vi "Get Dqmh Module Info.vi"(7 "Config":refnum<class "TAF Proj Config.lvclass">, 8 "error in":errorcluster, 11 "Library Ref":refnum<vi>) -> (0 "error out":errorcluster, 3 "Dqmh Module Info":T1={"Name"="", "Description"="", "Path"=path "", "Dqmh Module Type"=enum."Singleton", "Event Info"=[], "Start Module Info"={"Vi Path"=path "", "Name"="", "Description"="", "Event Type"=enum."Request", "Callers"=[], "Conpane Image"={"image type"=0, "image depth"=0, "image"=[], "mask"=[], "colors"=[], "Rectangle"={"left"=0, "top"=0, "right"=0, "bottom"=0}}}, "Stop Module Info"={"Vi Path"=path "", "Name"="", "Description"="", "Event Type"=enum."Request", "Callers"=[], "Conpane Image"={"image type"=0, "image depth"=0, "image"=[], "mask"=[], "colors"=[], "Rectangle"={"left"=0, "top"=0, "right"=0, "bottom"=0}}}, "Registred Broadcast"=[], "Custom Errors"=[], "Used Requests"=[], "Used Requests With Reply"=[]})   [LabVIEW 2021, in "TAF Proj Document Type.lvlib" / "Project Parser.lvlib"]
uses:
  <vilib>/Wovalab/AntiDoc/Document Type/Add-ons/LabVIEW TAF Project/Project Parser/Project Parser.lvlib
  <vilib>/Wovalab/AntiDoc/Document Type/Add-ons/LabVIEW TAF Project/Project Parser/Dqmh Module Info--cluster.ctl
  <vilib>/Wovalab/AntiDoc/Document Type/Add-ons/LabVIEW TAF Project/Project Parser/Dqmh Module Type--enum.ctl
  <vilib>/Wovalab/AntiDoc/Document Type/Add-ons/LabVIEW TAF Project/Project Parser/Dqmh Event Info--cluster.ctl
  <vilib>/Wovalab/AntiDoc/Document Type/Add-ons/LabVIEW TAF Project/Project Parser/Dqmh Event Type--enum.ctl
  <vilib>/Wovalab/AntiDoc/Document Type/Add-ons/LabVIEW TAF Project/Project Parser/Dqmh Event Links--cluster.ctl
  <vilib>/picture/picture.llb/imagedata.ctl
  <vilib>/Wovalab/AntiDoc/Document Type/Add-ons/LabVIEW TAF Project/Project Parser/Module Fonctions--cluster.ctl
  <vilib>/Wovalab/AntiDoc/Document Type/Add-ons/LabVIEW TAF Project/Project Parser/Custom Error Info.ctl
  <vilib>/Wovalab/AntiDoc/Document Type/Add-ons/LabVIEW TAF Project/Dqmh Module/Requests Used By Module--cluster.ctl
  <vilib>/Wovalab/AntiDoc/Document Type/Add-ons/LabVIEW TAF Project/TAF Proj Config/TAF Proj Config.lvclass
  <vilib>/Wovalab/AntiDoc/Document Type/Add-ons/LabVIEW TAF Project/Project Parser/Module Fonctions--enum.ctl
  <vilib>/Wovalab/AntiDoc/Document Type/Add-ons/LabVIEW TAF Project/Dqmh Module/Dqmh Module.lvclass
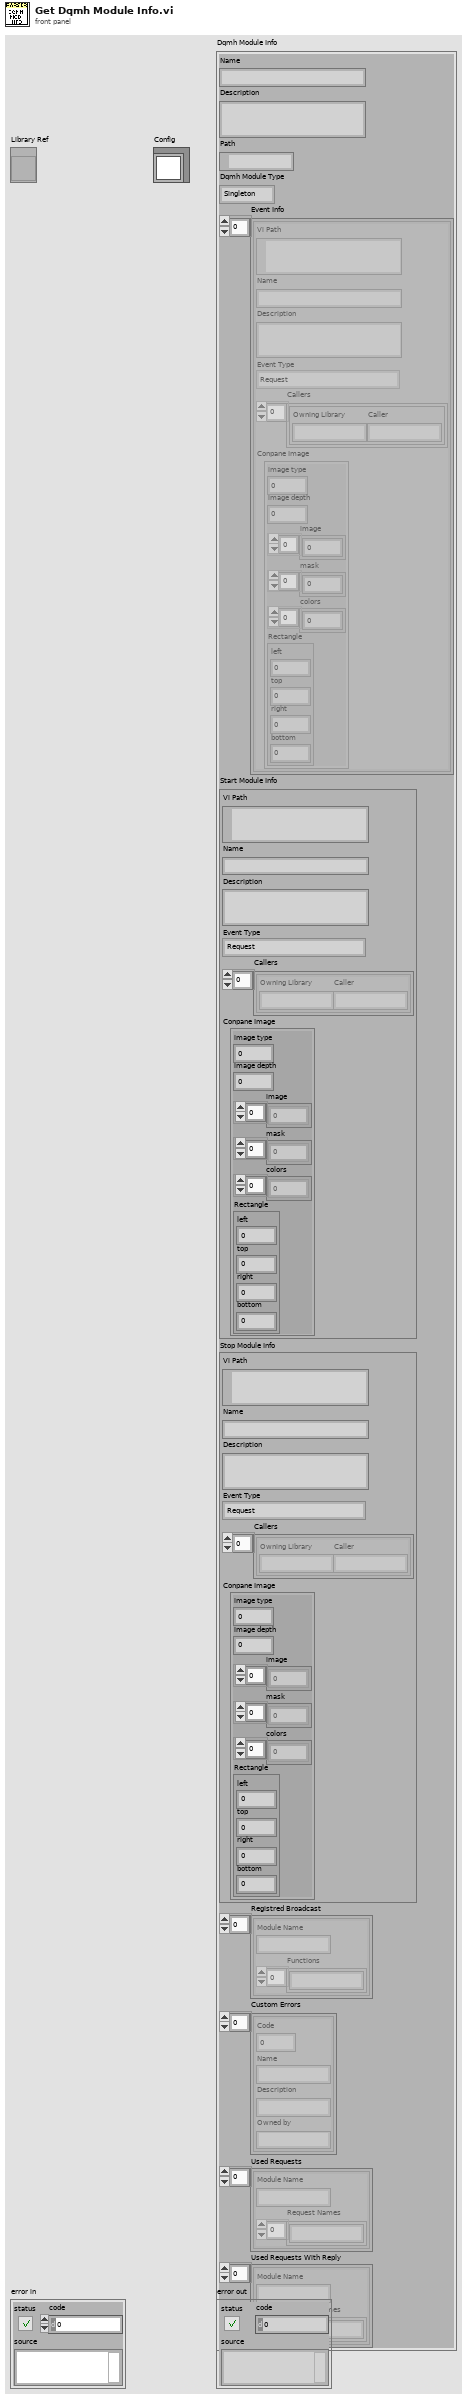
[diagram p1: front panel]
types:
  T1 = typedef "TAF Proj Document Type.lvlib/Project Parser.lvlib/Dqmh Module Info--cluster.ctl" = cluster{"Name":string, "Description":string, "Path":path, "Dqmh Module Type":T2, "Event Info":T3[], "Start Module Info":T3, "Stop Module Info":T3, "Registred Broadcast":T7[], "Custom Errors":T8[], "Used Requests":T9[], "Used Requests With Reply":T9[]}
  T2 = typedef "TAF Proj Document Type.lvlib/Project Parser.lvlib/Dqmh Module Type--enum.ctl" = enum16{"Singleton", "Cloneable"}
  T3 = typedef "TAF Proj Document Type.lvlib/Project Parser.lvlib/Dqmh Event Info--cluster.ctl" = cluster{"Vi Path":path, "Name":string, "Description":string, "Event Type":T4, "Callers":T5[], "Conpane Image":T6}
  T4 = typedef "TAF Proj Document Type.lvlib/Project Parser.lvlib/Dqmh Event Type--enum.ctl" = enum16{"Not a DQMH Event", "Request", "Request And Wait For Reply", "Broadcast"}
  T5 = typedef "TAF Proj Document Type.lvlib/Project Parser.lvlib/Dqmh Event Links--cluster.ctl" = cluster{"Owning Library":string, "Caller":string}
  T6 = typedef "imagedata.ctl" = cluster{"image type":i32, "image depth":i32, "image":u8[], "mask":u8[], "colors":u32[], "Rectangle":cluster{"left":i16, "top":i16, "right":i16, "bottom":i16}}
  T7 = typedef "TAF Proj Document Type.lvlib/Project Parser.lvlib/Module Fonctions--cluster.ctl" = cluster{"Module Name":string, "Functions":string[]}
  T8 = typedef "TAF Proj Document Type.lvlib/Project Parser.lvlib/Custom Error Info.ctl" = cluster{"Code":i32, "Name":string, "Description":string, "Owned by":string}
  T9 = typedef "TAF Proj Document Type.lvlib/Dqmh Module.lvclass/Requests Used By Module--cluster.ctl" = cluster{"Module Name":string, "Request Names":string[]}
  T10 = typedef "TAF Proj Document Type.lvlib/Project Parser.lvlib/Module Fonctions--enum.ctl" = enum16{"Event Registration", "Request"}
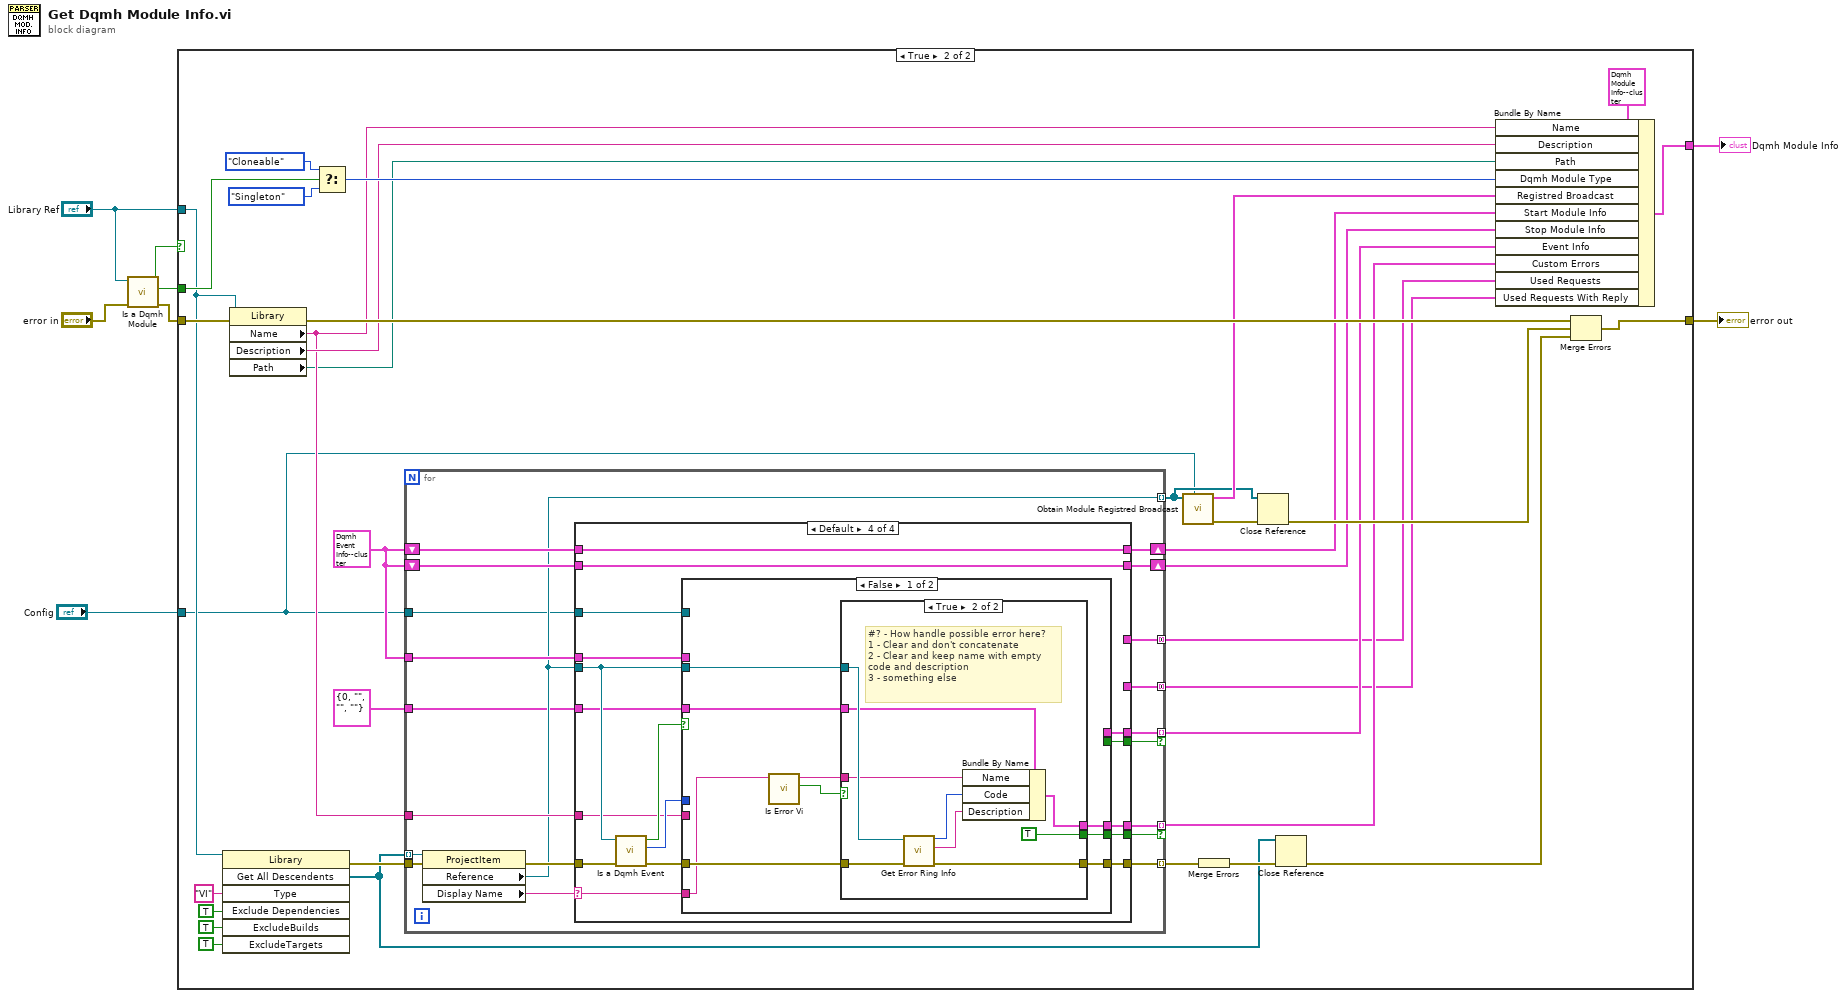
[diagram p0: block diagram]
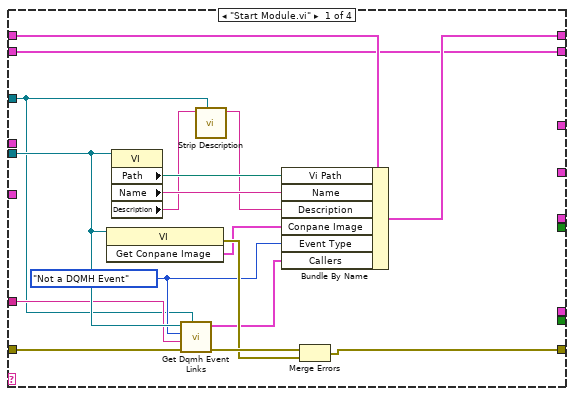
[diagram p3: hidden frame]
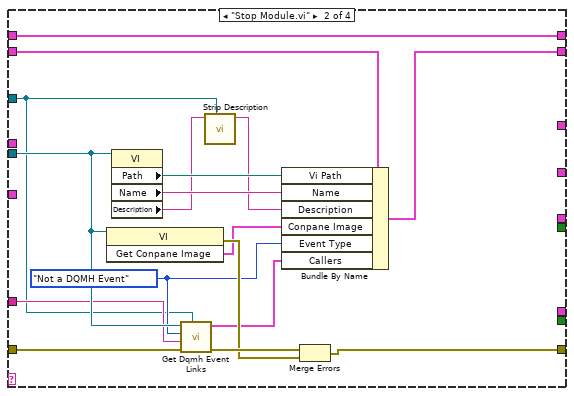
[diagram p4: hidden frame]
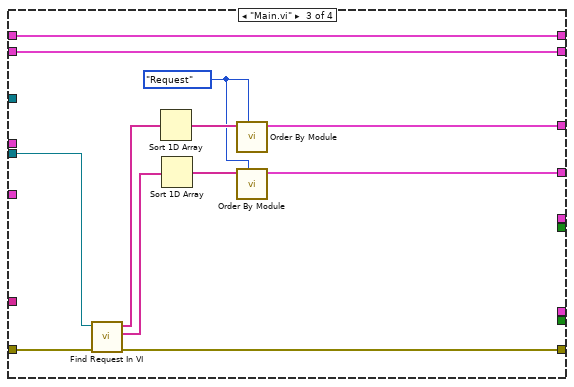
[diagram p5: hidden frame]
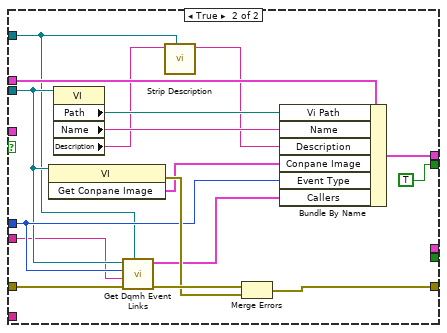
[diagram p7: hidden frame]
diagram:
  n1 = call <vilib>:"Is a Dqmh Module.vi"("error in"="error in", "Library Ref"="Library Ref") -> ("error out"=w6:errorcluster, "Is Cloneable"=w4:bool, "Is Dqmh Module"=w2:bool)  [unwired: 7 in]
  n2 = case shown="True" w2 {
    tunnel: [_ w35] -> w5
    tunnel: w4 -> [_ w34]
    tunnel: "Library Ref" -> [_ w29]
    tunnel: [w9 w41] -> w7
    tunnel: w6 -> [w9 w44]
    tunnel: "Config" -> [_ w12]
    frame False {
    }
    frame True {
      w21 = T3 {"Vi Path"=path "", "Name"="", "Description"="", "Event Type"=enum."Not a DQMH Event", "Callers"=[], "Conpane Image"={"image type"=0, "image depth"=0, "image"=[], "mask"=[], "colors"=[], "Rectangle"={"left"=0, "top"=0, "right"=0, "bottom"=0}}} ("Dqmh Event Info")
      n3 = invoke class="Library" method="Get All Descendents"(reference=w29, "Type"="VI", "Exclude Dependencies"=TRUE ("ExcludeDependencies"), "ExcludeBuilds"=TRUE, "ExcludeTargets"=TRUE) -> (error out=w43:errorcluster, "All Descendents"=w13:refnum<vi>[])  [unwired: 2 in, 5 out]
      n4 = property class="Library"(reference=w29, error in=w44) -> (error out=w42:errorcluster, "Name"=w22:string, "Description"=w30:string, "Path"=w17:path)  [unwired: 1 out]
      n5 = Select(t=Dqmh_Module_Type--enum."Cloneable" ("Dqmh Module Type"), s=w34, f=Dqmh_Module_Type--enum."Singleton") -> (s? t:f=w32:T2)
      n6 = for {
        tunnel: w13 -> [w58] mode=indexing
        tunnel: w21 -> [w61]
        tunnel: [w60] -> w27 mode=indexing if=w59
        tunnel: w43 -> [w63]
        tunnel: [w62] -> w26 mode=indexing
        tunnel: w22 -> [w57]
        shift-right: [w53] -> w19
        shift-left: w21 -> [w52]
        shift-right: [w55] -> w20
        shift-left: w21 -> [w54]
        tunnel: [w51] -> w14 mode=indexing
        tunnel: T8 {"Code"=0, "Name"="", "Description"="", "Owned by"=""} ("Custom Error Info") -> [w50]
        tunnel: [w49] -> w15 mode=indexing if=w48
        tunnel: w12 -> [w47]
        tunnel: [w46] -> w11 mode=concatenating
        tunnel: [w45] -> w10 mode=concatenating
        n7 = property class="ProjectItem"(reference=w58, error in=w63) -> (error out=w64:errorcluster, "Reference"=w51:refnum<vi>, "Display Name"=w56:string)  [unwired: 1 out]
        n8 = case shown="Default" w56 {
          selector: w56 -> [_ _ _ w115]
          tunnel: w64 -> [w79 w96 w106 w127]
          tunnel: [w78 w95 w107 w125] -> w62
          tunnel: w61 -> [_ _ _ w124]
          tunnel: [_ _ _ w121] -> w60
          tunnel: [_ _ _ w120] -> w59
          tunnel: w51 -> [w76 w94 w108 w119]
          tunnel: w57 -> [w71 w90 _ w118]
          tunnel: w54 -> [w77 w86 w110 w116]
          tunnel: [w72 w86 w110 w116] -> w55
          tunnel: [w69 w87 w109 w117] -> w53
          tunnel: w52 -> [w69 w88 w109 w117]
          tunnel: w50 -> [_ _ _ w114]
          tunnel: [_ _ _ w113] -> w49
          tunnel: [_ _ _ w112] -> w48
          tunnel: w47 -> [w65 w82 _ w111]
          tunnel: [_ _ w100 _] -> w46
          tunnel: [_ _ w99 _] -> w45
          frame "Start Module.vi" {
            w70 = Dqmh_Event_Type--enum."Not a DQMH Event" ("Event Type")
            n9 = invoke class="VI" method="Get Conpane Image"(reference=w76) -> (error out=w80:errorcluster, "Get Conpane Image"=w73:T6)  [unwired: 2 in, 1 out]
            n10 = property class="VI"(reference=w76) -> ("Path"=w75:path, "Name"=w68:string, "Description"=w67:string)  [unwired: 1 in, 2 out]
            n11 = call <vilib>:"Get Dqmh Event Links.vi"("Config"=w65, "error in"=w79, "Module Name"=w71, "Event Type"=w70, "VI Refnum"=w76) -> ("error out"=w81:errorcluster, "Links"=w74:T5[])  [unwired: 5 in]
            n12 = call <vilib>:"Strip Description.vi"("Config"=w65, "Description in"=w67) -> ("Description out"=w66:string)  [unwired: 9 in]
            n13 = Bundle By Name(cluster=w77, "Vi Path"=w75, "Name"=w68, "Description"=w66, "Conpane Image"=w73, "Event Type"=w70, "Callers"=w74) -> (w72:T3)
            n14 = Merge Errors(w81, w80) -> (w78:errorcluster)
          }
          frame "Stop Module.vi" {
            w89 = Dqmh_Event_Type--enum."Not a DQMH Event" ("Event Type")
            n15 = invoke class="VI" method="Get Conpane Image"(reference=w94) -> (error out=w97:errorcluster, "Get Conpane Image"=w91:T6)  [unwired: 2 in, 1 out]
            n16 = property class="VI"(reference=w94) -> ("Path"=w93:path, "Name"=w85:string, "Description"=w84:string)  [unwired: 1 in, 2 out]
            n17 = call <vilib>:"Get Dqmh Event Links.vi"("Config"=w82, "error in"=w96, "Module Name"=w90, "Event Type"=w89, "VI Refnum"=w94) -> ("error out"=w98:errorcluster, "Links"=w92:T5[])  [unwired: 5 in]
            n18 = call <vilib>:"Strip Description.vi"("Config"=w82, "Description in"=w84) -> ("Description out"=w83:string)  [unwired: 9 in]
            n19 = Bundle By Name(cluster=w88, "Vi Path"=w93, "Name"=w85, "Description"=w83, "Conpane Image"=w91, "Event Type"=w89, "Callers"=w92) -> (w87:T3)
            n20 = Merge Errors(w98, w97) -> (w95:errorcluster)
          }
          frame "Main.vi" {
            w101 = Module_Fonctions--enum."Request" ("Mode")
            n21 = call <vilib>:"Find Request In VI.vi"("error in"=w106, "VI Ref"=w108) -> ("error out"=w107:errorcluster, "Request And Wait For Reply Names"=w103:string[], "Request Names"=w105:string[])  [unwired: 6 in, 1 out]
            n22 = Sort 1D Array(array=w105) -> (sorted array=w104:string[])
            n23 = Sort 1D Array(array=w103) -> (sorted array=w102:string[])
            n24 = call <vilib>:"Order By Module.vi"("Mode"=w101, "Functions"=w104) -> ("Functions by Module"=w100:T7[])  [unwired: 9 in]
            n25 = call <vilib>:"Order By Module.vi"("Mode"=w101, "Functions"=w102) -> ("Functions by Module"=w99:T7[])  [unwired: 9 in]
          }
          frame Default {
            n26 = call <vilib>:"Is a Dqmh Event.vi"("error in"=w127, "VI Refnum"=w119) -> ("error out"=w126:errorcluster, "Event Type"=w123:T4, "Is Dqmh Event"=w122:bool)  [unwired: 7 in]
            n27 = case shown="False" w122 {
              tunnel: w124 -> [_ w159]
              tunnel: w123 -> [_ w154]
              tunnel: w119 -> [w132 w153]
              tunnel: [_ w157] -> w121
              tunnel: [_ TRUE] -> w120
              tunnel: w126 -> [w135 w163]
              tunnel: [w136 w161] -> w125
              tunnel: w118 -> [_ w151]
              tunnel: w115 -> [w134 _]
              tunnel: w114 -> [w130 _]
              tunnel: [w129 _] -> w113
              tunnel: [w128 _] -> w112
              tunnel: w111 -> [_ w147]
              frame False {
                n28 = call <vilib>:"Is Error Vi.vi"("Vi Name"=w134) -> ("Error Vi?"=w133:bool, "Error Name"=w131:string)  [unwired: 9 in]
                n29 = case shown="True" w133 {
                  tunnel: [w137 w145] -> w136
                  tunnel: w135 -> [w137 w146]
                  tunnel: w132 -> [_ w144]
                  tunnel: w131 -> [_ w141]
                  tunnel: w130 -> [_ w143]
                  tunnel: [_ w142] -> w129
                  tunnel: [_ TRUE] -> w128
                  frame False {
                  }
                  frame True {
                    # "#? - How handle possible error here?\n1 - Clear and don't concatenate\n2 - Clear and keep name with empty code and description\n3 - something else"
                    n30 = call <vilib>:"Get Error Ring Info.vi"("error in"=w146, "Error VI Refnum"=w144) -> ("error out"=w145:errorcluster, "Custom Description"=w139:string, "code"=w140:i32)  [unwired: 7 in]
                    n31 = Bundle By Name(cluster=w143, "Name"=w141, "Code"=w140, "Description"=w139) -> (w142:T8)
                  }
                }
              }
              frame True {
                n32 = invoke class="VI" method="Get Conpane Image"(reference=w153) -> (error out=w160:errorcluster, "Get Conpane Image"=w152:T6)  [unwired: 2 in, 1 out]
                n33 = property class="VI"(reference=w153) -> ("Path"=w158:path, "Name"=w150:string, "Description"=w149:string)  [unwired: 1 in, 2 out]
                n34 = call <vilib>:"Get Dqmh Event Links.vi"("Config"=w147, "error in"=w163, "Module Name"=w151, "Event Type"=w154, "VI Refnum"=w153) -> ("error out"=w162:errorcluster, "Links"=w155:T5[])  [unwired: 5 in]
                n35 = call <vilib>:"Strip Description.vi"("Config"=w147, "Description in"=w149) -> ("Description out"=w148:string)  [unwired: 9 in]
                n36 = Merge Errors(w162, w160) -> (w161:errorcluster)
                n37 = Bundle By Name(cluster=w159, "Vi Path"=w158, "Name"=w150, "Description"=w148, "Conpane Image"=w152, "Event Type"=w154, "Callers"=w155) -> (w157:T3)
              }
            }
          }
        }
      }
      n38 = call <vilib>:"Obtain Module Registred Broadcast.vi"("Config"=w12, "VI References"=w14) -> ("error out"=w40:errorcluster, "Registred Broadcast"=w18:T7[])  [unwired: 8 in]
      n39 = Merge Errors(w26) -> (w38:errorcluster)
      n40 = Close Reference(reference=w14, error in (no error)=w40) -> (error out=w39:errorcluster)
      n41 = Close Reference(reference=w13, error in (no error)=w38) -> (error out=w37:errorcluster)
      n42 = Bundle By Name(cluster=T1 {"Name"="", "Description"="", "Path"=path "", "Dqmh Module Type"=enum."Singleton", "Event Info"=[], "Start Module Info"={"Vi Path"=path "", "Name"="", "Description"="", "Event Type"=enum."Request", "Callers"=[], "Conpane Image"={"image type"=0, "image depth"=0, "image"=[], "mask"=[], "colors"=[], "Rectangle"={"left"=0, "top"=0, "right"=0, "bottom"=0}}}, "Stop Module Info"={"Vi Path"=path "", "Name"="", "Description"="", "Event Type"=enum."Request", "Callers"=[], "Conpane Image"={"image type"=0, "image depth"=0, "image"=[], "mask"=[], "colors"=[], "Rectangle"={"left"=0, "top"=0, "right"=0, "bottom"=0}}}, "Registred Broadcast"=[], "Custom Errors"=[], "Used Requests"=[], "Used Requests With Reply"=[]} ("Dqmh Module Info"), "Name"=w22, "Description"=w30, "Path"=w17, "Dqmh Module Type"=w32, "Registred Broadcast"=w18, "Start Module Info"=w20, "Stop Module Info"=w19, "Event Info"=w27, "Custom Errors"=w15, "Used Requests"=w11, "Used Requests With Reply"=w10) -> (w35:T1)
      n43 = Merge Errors(w42, w39, w37) -> (w41:errorcluster)
    }
  }
  "Dqmh Module Info" <- w5
  "error out" <- w7
